vi "test_Add Command_Variable Number Error.vi"(8 "error in (no error)":errorcluster, 11 "TestCase in":refnum<class "Instrument Addon Scripting API Messages Unit Tests.lvclass">) -> (0 "error out":errorcluster, 3 "TestCase out":refnum<class "Instrument Addon Scripting API Messages Unit Tests.lvclass">)   [LabVIEW 2019, in "Instrument Addon Scripting API Messages Unit Tests.lvclass"]
uses:
  Instrument Addon Scripting API Messages Unit Tests.lvclass
  APIs/Scripting API/TypeDefs/Command Settings.ctl
  <vilib>/NI VeriStand/Custom Device API/Custom Device Item Ref.ctl
  APIs/Scripting API/TypeDefs/Padding.ctl
  Instrument Addon Scripting API Messages Unit Tests.lvclass/Instrument Addon Scripting API Messages Unit Tests.ctl
  Addon/Addon Shared/SubVIs/Constants.vi
  <vilib>/NI/NI VeriStand Advanced SysDef API/_SubVIs/SysDef.Search.GUID.vi
  <vilib>/addons/_JKI Toolkits/VI Tester/TestCase.llb/TestCase.lvclass
  <vilib>/NI/NI VeriStand Advanced SysDef API/SysDef API/Advanced System Definition.lvlib
  Addon/Addon Shared/Instrument Addon Shared.lvlib
  <vilib>/NI VeriStand/Custom Device API/Custom Device API.lvlib
  APIs/Scripting API/Instrument Addon Scripting API.lvlib
  C:/Program Files (x86)/National Instruments/LabVIEW 2019/vi.lib/addons/_JKI Toolkits/VI Tester/TestCase.llb/TestCase.lvclass
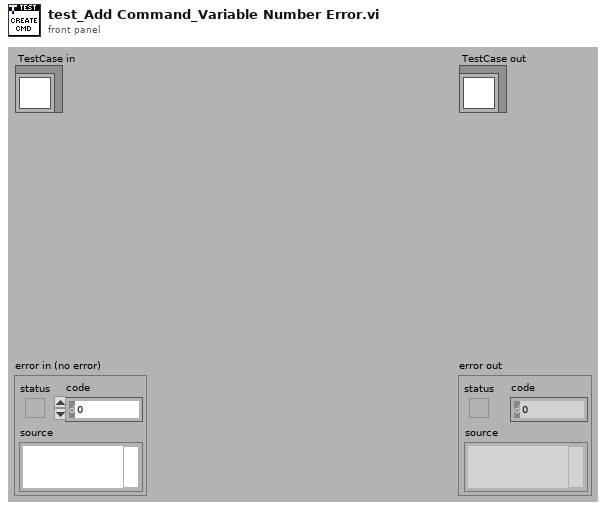
[diagram p1: front panel]
types:
  T1 = typedef "Instrument Addon Scripting API.lvlib/Command Settings.ctl" = cluster{"Command Format":string, "Linked Channels":cluster{"Variable Name":string, "Channel Ref in":T2}[], "Use Padding?":bool, "Padding":T3}
  T2 = typedef "Custom Device API.lvlib/Custom Device Item Ref.ctl" = u64
  T3 = typedef "Instrument Addon Scripting API.lvlib/Padding.ctl" = cluster{"Pad Value":u8, "Length":u32}
  T4 = typedef "Instrument Addon Scripting API.lvlib/Linked Channel.ctl" = cluster{"Variable Name":string, "Channel Refnum":T2}
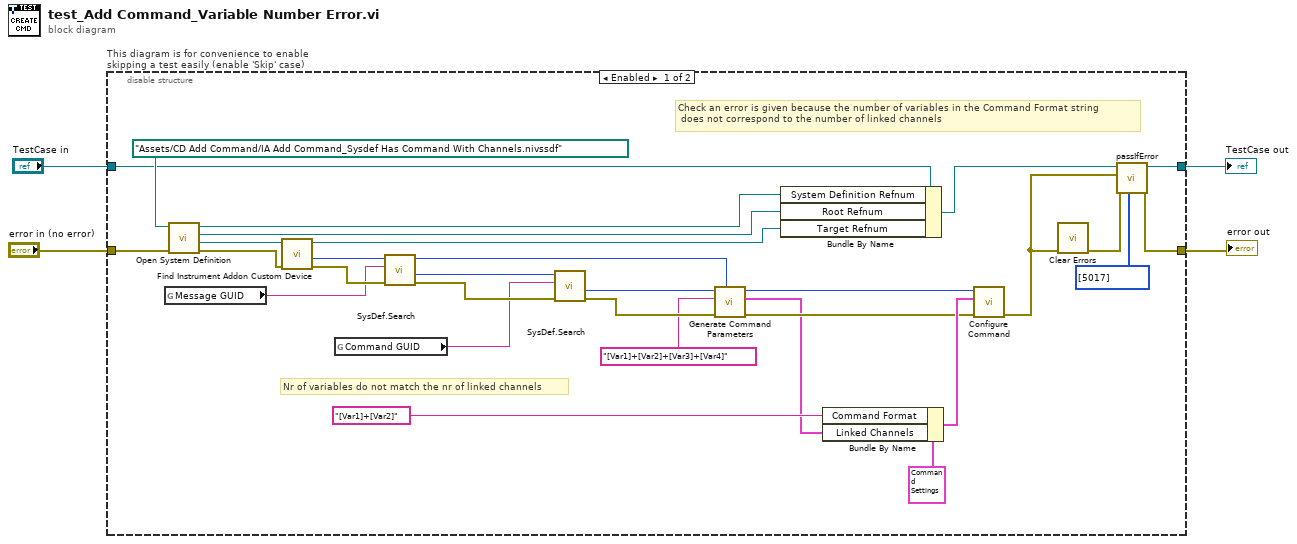
[diagram p0: block diagram]
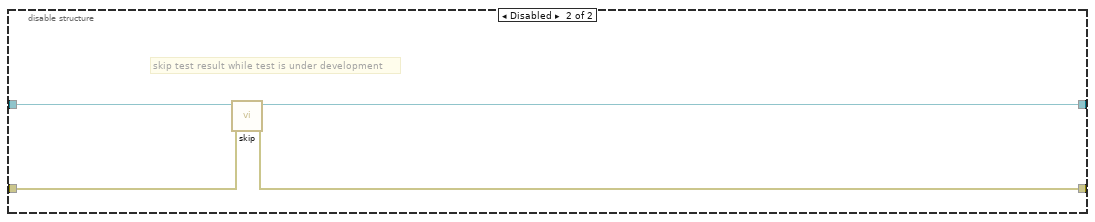
[diagram p2: hidden frame]
diagram:
  n1 = disable-structure "This diagram is for convenience to enable skipping a test easily (enable 'Skip' case)" shown="Enabled" {
    disable-tunnel: "TestCase in" -> [w21 w38]
    disable-tunnel: [w31 w36] -> w1
    disable-tunnel: [w32 w37] -> w3
    disable-tunnel: "error in (no error)" -> [w33 w35]
    frame Enabled {
      # "Nr of variables do not match the nr of linked channels"
      # "Check an error is given because the number of variables in the Command Format string\n does not correspond to the number of linked channels"
      n2 = global read "Constants.vi" "Message GUID"() -> (w27:string)
      n3 = call "Open System Definition.vi"("error in (no error)"=w33, "System Definition File"=path "Assets/CD Add Command/IA Add Command_Sysdef Has Command With Channels.nivssdf" ("SDF file")) -> ("error out"=w29:errorcluster, "Target Refnum"=w30:refnum<k24>, "Root Refnum"=w18:refnum<k24>, "System Definition Refnum"=w19:refnum<k24>)  [unwired: 6 in]
      n4 = call "Find Instrument Addon Custom Device.vi"("error in"=w29, "target in"=w30) -> ("error out"=w28:errorcluster, "NodeID"=w24:u64, "target out"=w17:refnum<k24>)  [unwired: 7 in]
      n5 = global read "Constants.vi" "Command GUID"() -> (w12:string)
      n6 = call-poly <vilib>:"SysDef.Search.vi"("error in (no error)"=w28, "GUID"=w27, "nodeID"=w24) -> ("error out"=w13:errorcluster, "Value out"=w14:u64, "nodeID out"=w5:u64)  [unwired: 5 in, 1 out]
      n7 = call-poly <vilib>:"SysDef.Search.vi"("error in (no error)"=w13, "GUID"=w12, "nodeID"=w14) -> ("error out"=w9:errorcluster, "Value out"=w11:u64)  [unwired: 5 in, 2 out]
      n8 = call "Generate Command Parameters.vi"("Instrument Addon Refnum in"=w5, "Error In"=w9, "Command String"="[Var1]+[Var2]+[Var3]+[Var4]" ("Command Format"), "Command Channel in"=w11) -> ("Error Out"=w8:errorcluster, "Linked Channels"=w6:T4[], "Command Channel out"=w10:T2)  [unwired: 4 in, 1 out]
      n9 = Bundle By Name(cluster=w21, "System Definition Refnum"=w19, "Root Refnum"=w18, "Target Refnum"=w17) -> (w20:refnum<class "Instrument Addon Scripting API Messages Unit Tests.lvclass">)
      n10 = Bundle By Name(cluster=T1 {"Command Format"="[Var1]+[Var2]", "Linked Channels"=[{"Variable Name"="Var1", "Channel Ref in"=32}, {"Variable Name"="Var2", "Channel Ref in"=33}], "Use Padding?"=FALSE, "Padding"={"Pad Value"=0, "Length"=0}} ("Settings"), "Command Format"="[Var1]+[Var2]", "Linked Channels"=w6) -> (w15:T1)
      n11 = call "Configure Command.vi"("error in (no error)"=w8, "settings"=w15, "command refnum in"=w10) -> ("error out"=w16:errorcluster)  [unwired: 7 in, 1 out]
      n12 = call <vilib>:"Clear Errors.vi"("error in (no error)"=w16) -> ("error out"=w22:errorcluster)  [unwired: 5 in, 1 out]
      n13 = call-dynamic "passIfError.vi"("passing error codes (default = any error code)"=i32[] [5017], "error in (no error)"=w22, "error"=w16, "TestCase in"=w20) -> ("error out"=w32:errorcluster, "TestCase out"=w31:refnum<class "Instrument Addon Scripting API Messages Unit Tests.lvclass">)  [unwired: 6 in]
    }
    frame Disabled {
      # "skip test result while test is under development"
      n14 = call <vilib>:"skip.vi"("error in (no error)"=w35, "TestCase in"=w38) -> ("error out"=w37:errorcluster, "TestCase out"=w36:refnum<class "Instrument Addon Scripting API Messages Unit Tests.lvclass">)  [unwired: 8 in]
    }
  }
  "error out" <- w3
  "TestCase out" <- w1
